vi "20211015_01.vi"() -> ()   [LabVIEW 2019]
panel:
  out "Filename":string
  in  "File Path":path
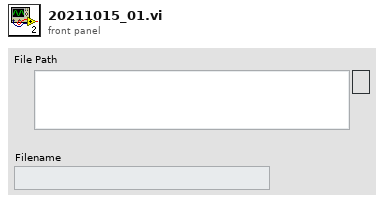
[diagram p1: front panel]
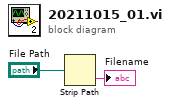
[diagram p0: block diagram]
diagram:
  n1 = Strip Path(path="File Path") -> (name=→"Filename":string)  [unwired: 1 out]
